vi "WPI_RobotDriveOpen2Wheel.vi"   [LabVIEW 2019]
doc: "Opens a reference to the motors you indicate and specifies the responsiveness of the joystick to the motors. You must open a reference before using any other VIs on this palette.\n\nThis software is licensed. Open the labview\\readme\\WPI Robotics Library Open Source License.txt file for more information."
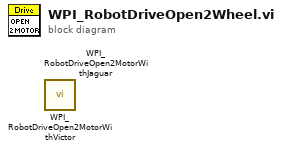
[diagram p0: block diagram]
diagram:
  n1 = call <vilib>:"WPI_RobotDriveOpen2MotorWithVictor.vi"() -> ()  [unwired: 10 in, 2 out]
  n2 = call <vilib>:"WPI_RobotDriveOpen2MotorWithJaguar.vi"() -> ()  [unwired: 10 in, 2 out]
